vi "Exp no 6a Application of FOR LOOP.vi"() -> ()   [LabVIEW 2010]
panel:
  in  "N":i32
  out "Sum of N Natural Numbers":i32[](array[numeric])
  # "SUM OF N NATURAL NUMBERS"
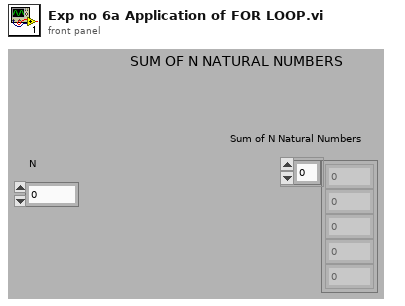
[diagram p1: front panel]
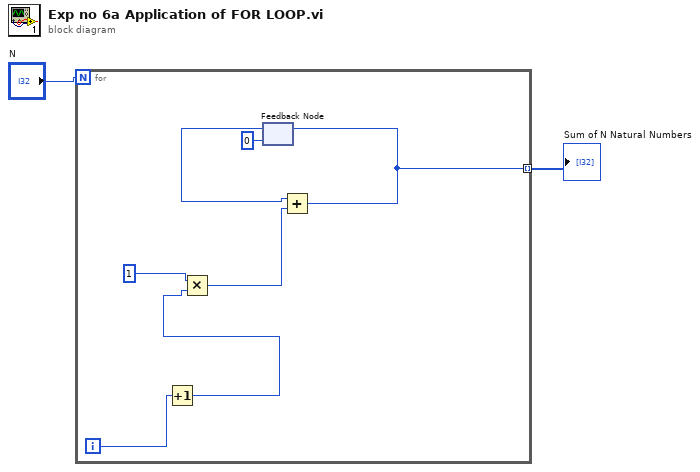
[diagram p0: block diagram]
diagram:
  n1 = for {
    N: "N" -> [_]
    tunnel: [w3] -> w2 mode=indexing
    i -> [w9]
    n2 = Increment(x=w9) -> (x+1=w8:i32)
    n3 = Multiply(x=1, y=w8) -> (x*y=w6:i32)
    n4 = feedback #1(0) -> (w5:i32)
    n5 = Add(x=w5, y=w6) -> (x+y=w3:i32)
    n6 = feedback-in #1(w3) -> ()
  }
  "Sum of N Natural Numbers" <- w2
